vi "setUp.vi"(7 "stop 2":bool, 8 "Sim/Live":bool, 9 "stop":bool) -> (0 "Ready":bool, 1 "SystemID":i32, 2 "Error Out":errorcluster, 3 "AxisID":string[](array[string]), 4 "AxisID 2":string[](array[string]), 5 "Ready 2":bool, 6 "SystemID 2":i32)   [LabVIEW 2019]
panel:
  in  "Error In":errorcluster
  out "STOP":bool
  # "LIVE"
  # "SIMULATION"
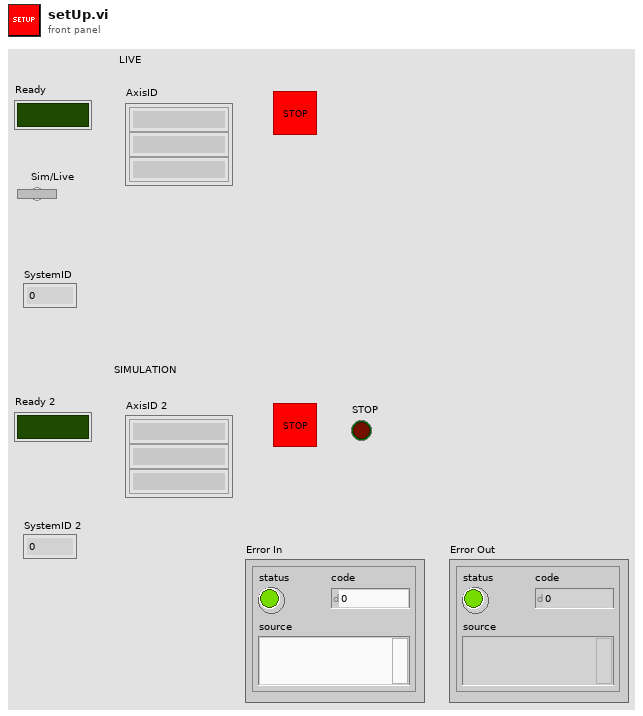
[diagram p1: front panel]
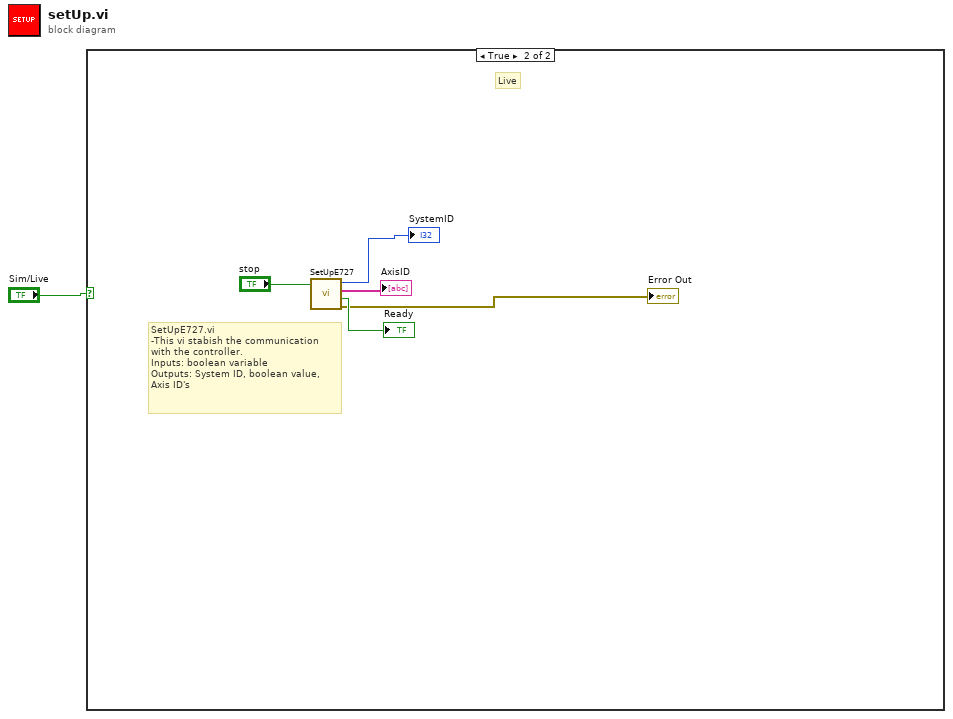
[diagram p0: block diagram]
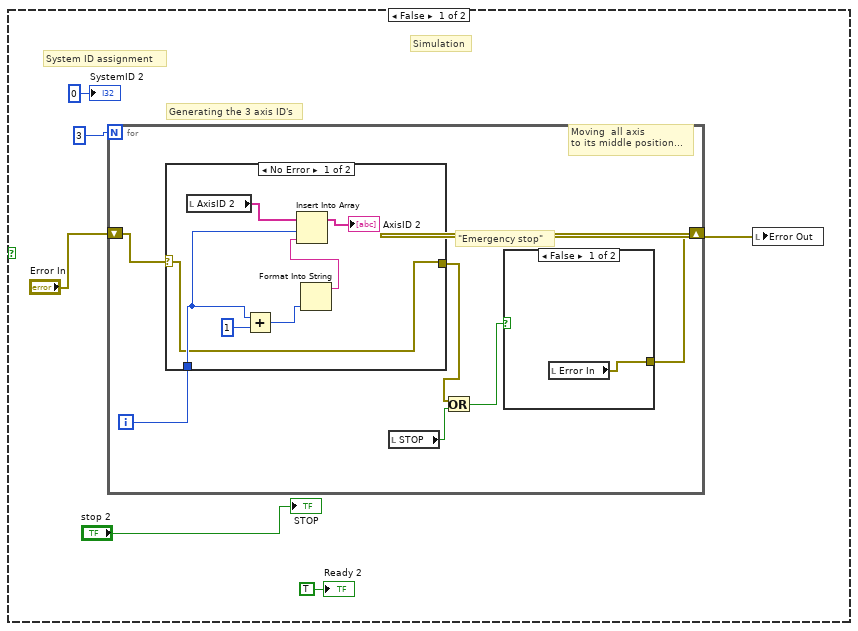
[diagram p2: hidden frame]
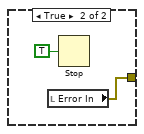
[diagram p3: hidden frame]
diagram:
  n1 = case shown="True" "Sim/Live" {
    frame False {
      # "Moving  all axis \nto its middle position..."
      # "System ID assignment"
      # "Generating the 3 axis ID's"
      # "Simulation"
      n2 = for {
        N: 3 -> [_]
        shift-right: [w8] -> w3
        shift-left: "Error In" -> [w12]
        i -> [w13]
        # "\"Emergency stop\""
        n3 = case shown="No Error" w12 {
          selector: w12 -> [w17 w24]
          tunnel: w13 -> [w19 _]
          tunnel: [w17 w24] -> w10
          frame No Error {
            n4 = local read "AxisID 2"() -> (w21:string[])
            n5 = Add(x=w19, y=1) -> (x+y=w20:i32)
            n6 = Format Into String(w20) -> (resulting string=w23:string)  [unwired: 3 in, 1 out]
            n7 = Insert Into Array(array=w21, index=w19, new element=w23) -> (→"AxisID 2":string[])
          }
          frame Error {
          }
        }
        n8 = local read "STOP"() -> (w11:bool)
        n9 = Or(x=w10, y=w11) -> (x .or. y?=w9:bool)
        n10 = case shown="False" w9 {
          tunnel: [w14 w15] -> w8
          frame False {
            n11 = local read "Error In"() -> (w14:errorcluster)
          }
          frame True {
            n12 = local read "Error In"() -> (w15:errorcluster)
            n13 = Stop(stop? (T)=TRUE) -> ()
          }
        }
      }
      n14 = local write "Error Out"(w3) -> ()
      "Ready 2" <- TRUE ("Ready 2")
      "SystemID 2" <- 0 ("SytemID 2")
      "STOP" <- "stop 2"
    }
    frame True {
      # "SetUpE727.vi\n-This vi stabish the communication \nwith the controller.\nInputs: boolean variable\nOutputs: System ID, boolean value,\nAxis ID's"
      # "Live"
      n15 = call "SetUpE727.vi"("stop"="stop") -> ("Error Out"=→"Error Out":errorcluster, "Redy"=→"Ready":bool, "Axis ID´s"=→"AxisID":string[], "SystemID"=→"SystemID":i32)  [unwired: 7 in]
    }
  }
